vi "ROI entry screen-Fit ROI to new frame size.vi"(9 "ROI fit info":T1 {"ROI fit info"."Frame size"."Old" items=["100X100"=100, "128X128"=128, "200X200"=200, "256X256"=256, "512X512"=512, "1024x1024"=1024, "2048x2048"=2048]; "ROI fit info"."Frame size"."New" items=["100X100"=100, "128X128"=128, "200X200"=200, "256X256"=256, "512X512"=512, "1024x1024"=1024, "2048x2048"=2048]}, 11 "Old ROI file's data in":dbl[][](array[numeric])) -> (3 "Old ROI file's data out":dbl[][](array[numeric]))   [LabVIEW 2017]
uses:
  Typedefs/ROI fitting info cluster.ctl
  Typedefs/Frame Size.ctl
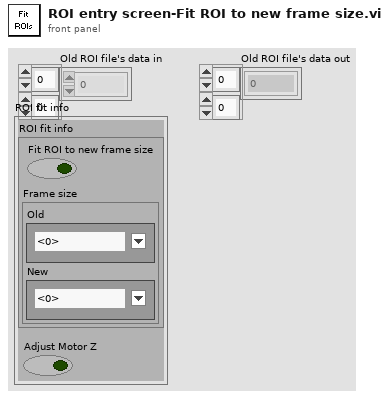
[diagram p1: front panel]
types:
  T1 = typedef "ROI fitting info cluster.ctl" = cluster{"ROI fit info":cluster{"Fit ROI to new frame size":bool, "Frame size":cluster{"Old":T2, "New":T2}}, "Adjust Motor Z":bool}
  T2 = typedef "Frame Size.ctl" = u16
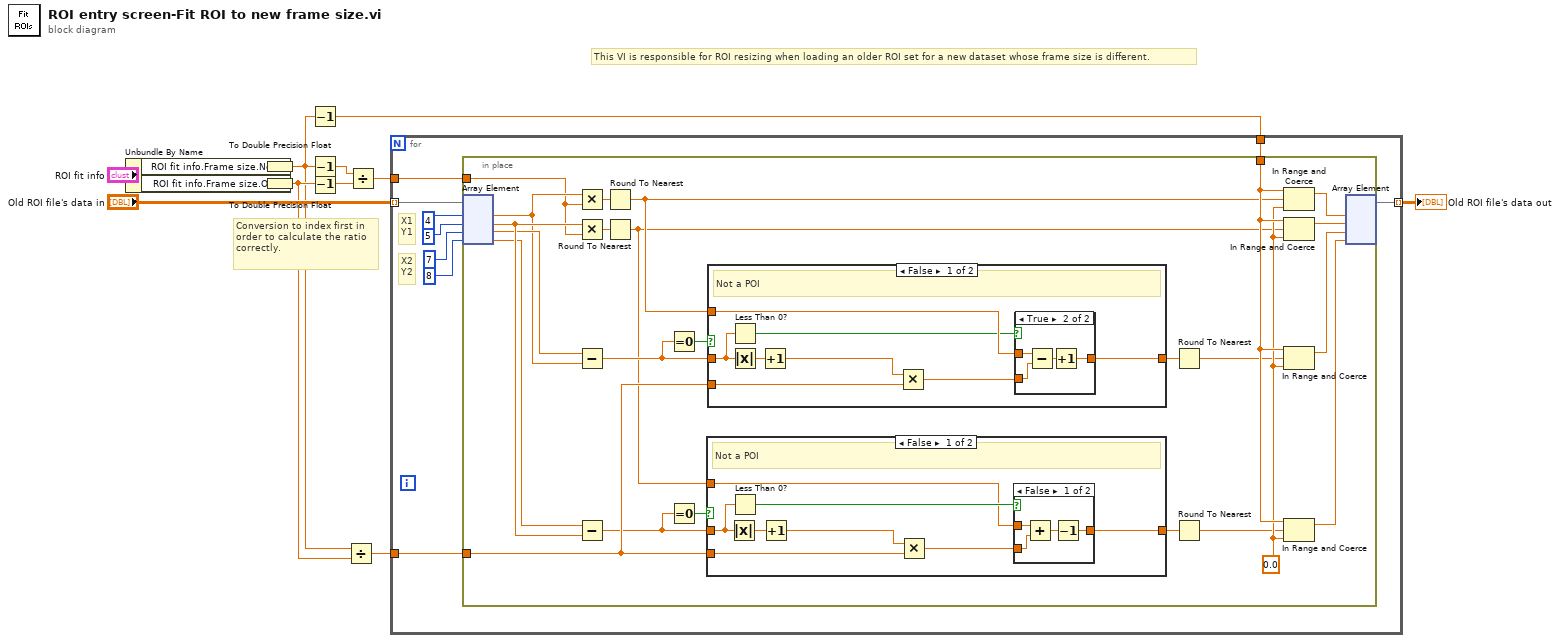
[diagram p0: block diagram]
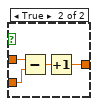
[diagram p2: hidden frame]
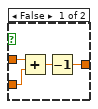
[diagram p4: hidden frame]
diagram:
  # "This VI is responsible for ROI resizing when loading an older ROI set for a new dataset whose frame size is different."
  # "Conversion to index first in order to calculate the ratio correctly."
  n1 = Unbundle By Name("ROI fit info") -> ("ROI fit info.Frame size.New"=w2:T2, "ROI fit info.Frame size.Old"=w3:T2)
  n2 = To Double Precision Float(number=w2) -> (double precision float=w8:dbl)
  n3 = To Double Precision Float(number=w3) -> (double precision float=w9:dbl)
  n4 = Decrement(x=w8) -> (x-1=w5:dbl)
  n5 = Decrement(x=w8) -> (x-1=w6:dbl)
  n6 = Decrement(x=w9) -> (x-1=w7:dbl)
  n7 = Divide(x=w8, y=w9) -> (x/y=w10:dbl)
  n8 = Divide(x=w6, y=w7) -> (x/y=w4:dbl)
  n9 = for {
    tunnel: "Old ROI file's data in" -> [w21] mode=indexing
    tunnel: w4 -> [w15]
    tunnel: [w16] -> w11 mode=indexing
    tunnel: w5 -> [w14]
    tunnel: w10 -> [w13]
    # "X2\nY2"
    # "X1\nY1"
    n10 = in-place {
      in-place-border: w15 -> [w29]
      in-place-border: w14 -> [w42]
      in-place-border: w13 -> [w28]
      w41 = 0.0 ("x-1")
      n11 = in-place-array #1(w21, 4 ("index"), 5 ("index"), 7 ("index"), 8 ("index")) -> (w30:dbl, w37:dbl, w35:dbl, w31:dbl)
      n12 = Multiply(x=w30, y=w29) -> (x*y=w44:dbl)
      n13 = Multiply(x=w37, y=w29) -> (x*y=w45:dbl)
      n14 = Subtract(x=w35, y=w30) -> (x-y=w27:dbl)
      n15 = Subtract(x=w31, y=w37) -> (x-y=w26:dbl)
      n16 = Round To Nearest(number=w44) -> (nearest integer value=w25:dbl)
      n17 = Round To Nearest(number=w45) -> (nearest integer value=w23:dbl)
      n18 = Equal To 0?(x=w27) -> (x = 0?=w36:bool)
      n19 = Equal To 0?(x=w26) -> (x = 0?=w32:bool)
      n20 = case shown="False" w32 {
        tunnel: [w48 w62] -> w33
        tunnel: w26 -> [w51 _]
        tunnel: w28 -> [w53 _]
        tunnel: w23 -> [w47 w62]
        frame False {
          # "Not a POI"
          n21 = Absolute Value(x=w51) -> (abs(x)=w52:dbl)
          n22 = Less Than 0?(x=w51) -> (x < 0?=w50:bool)
          n23 = Increment(x=w52) -> (x+1=w46:dbl)
          n24 = Multiply(x=w46, y=w53) -> (x*y=w49:dbl)
          n25 = case shown="False" w50 {
            tunnel: w47 -> [w57 w61]
            tunnel: w49 -> [w56 w60]
            tunnel: [w54 w58] -> w48
            frame False {
              n26 = Add(x=w57, y=w56) -> (x+y=w55:dbl)
              n27 = Decrement(x=w55) -> (x-1=w54:dbl)
            }
            frame True {
              n28 = Subtract(x=w61, y=w60) -> (x-y=w59:dbl)
              n29 = Increment(x=w59) -> (x+1=w58:dbl)
            }
          }
        }
        frame True {
          # "Ensures the resulting Y1 and Y2 are the same since\nPOI must have equal Y1 and Y2."
          # "POI"
        }
      }
      n30 = case shown="False" w36 {
        tunnel: [w68 w79] -> w34
        tunnel: w27 -> [w66 _]
        tunnel: w28 -> [w70 _]
        tunnel: w25 -> [w69 w79]
        frame False {
          # "Not a POI"
          n31 = Less Than 0?(x=w66) -> (x < 0?=w65:bool)
          n32 = Absolute Value(x=w66) -> (abs(x)=w67:dbl)
          n33 = Increment(x=w67) -> (x+1=w64:dbl)
          n34 = Multiply(x=w64, y=w70) -> (x*y=w63:dbl)
          n35 = case shown="True" w65 {
            tunnel: w69 -> [w74 w78]
            tunnel: w63 -> [w73 w77]
            tunnel: [w71 w75] -> w68
            frame False {
              n36 = Add(x=w74, y=w73) -> (x+y=w72:dbl)
              n37 = Decrement(x=w72) -> (x-1=w71:dbl)
            }
            frame True {
              n38 = Subtract(x=w78, y=w77) -> (x-y=w76:dbl)
              n39 = Increment(x=w76) -> (x+1=w75:dbl)
            }
          }
        }
        frame True {
          # "Ensures the resulting X1 and X2 are the same since\nPOI must have equal X1 and X2."
          # "POI"
        }
      }
      n40 = Round To Nearest(number=w34) -> (nearest integer value=w24:dbl)
      n41 = Round To Nearest(number=w33) -> (nearest integer value=w22:dbl)
      n42 = In Range and Coerce(upper limit=w42, x=w25, lower limit=w41) -> (coerced(x)=w43:dbl)  [unwired: 1 out]
      n43 = In Range and Coerce(upper limit=w42, x=w23, lower limit=w41) -> (coerced(x)=w40:dbl)  [unwired: 1 out]
      n44 = In Range and Coerce(upper limit=w42, x=w24, lower limit=w41) -> (coerced(x)=w39:dbl)  [unwired: 1 out]
      n45 = In Range and Coerce(upper limit=w42, x=w22, lower limit=w41) -> (coerced(x)=w38:dbl)  [unwired: 1 out]
      n46 = in-place-array #1(w43, w40, w39, w38) -> (w16:dbl[])  [unwired: 4 out]
    }
  }
  "Old ROI file's data out" <- w11
